vi "Active Graphic On Click.vi"(8 "error in (no error)":errorcluster, 10 "MousePoint":cluster{"x":i16, "y":i16}, 11 "Canvas in":refnum<class "Canvas.lvclass">) -> (0 "error out":errorcluster, 2 "Find?":bool, 3 "Canvas out":refnum<class "Canvas.lvclass">)   [LabVIEW 2015, in "Canvas.lvclass"]
uses:
  Canvas.lvclass
  Canvas.lvclass/Canvas.ctl
  Graphic/Graphic.lvclass
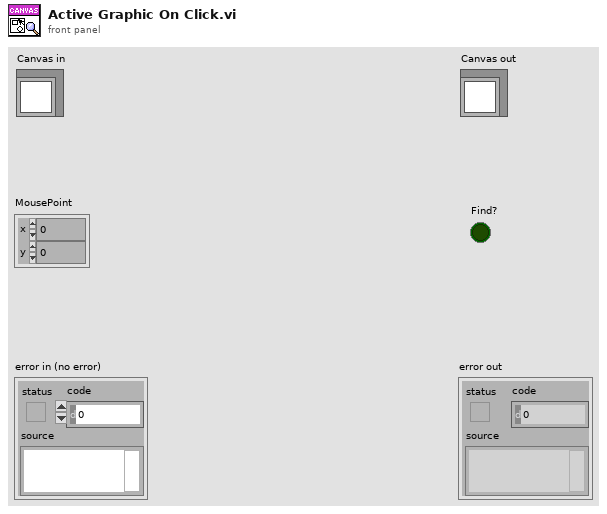
[diagram p1: front panel]
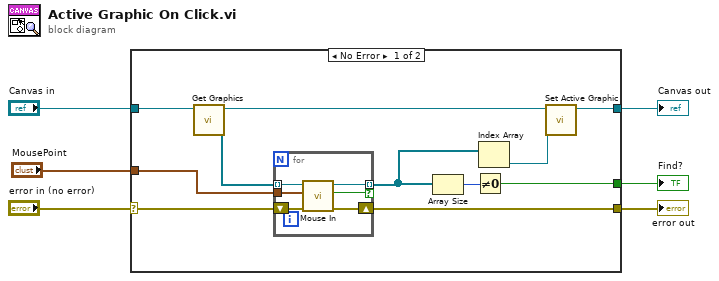
[diagram p0: block diagram]
diagram:
  n1 = case shown="No Error" "error in (no error)" {
    selector: "error in (no error)" -> [w13 w25]
    tunnel: [w12 w25] -> w5
    tunnel: [w8 w24] -> w3
    tunnel: "Canvas in" -> [w17 w24]
    tunnel: "MousePoint" -> [w14 _]
    tunnel: [w9 _] -> w1
    frame No Error {
      n2 = call "Get Graphics.vi"("Canvas in"=w17) -> ("Graphics"=w15:refnum<class "Graphic.lvclass">[], "Canvas out"=w16:refnum<class "Canvas.lvclass">)  [unwired: 8 in, 1 out]
      n3 = for {
        tunnel: w15 -> [w23] mode=indexing
        tunnel: w14 -> [w22]
        shift-right: [w20] -> w12
        shift-left: w13 -> [w21]
        tunnel: [w19] -> w11 mode=indexing if=w18
        n4 = call-dynamic "Mouse In.vi"("error in (no error)"=w21, "MousePoint"=w22, "Graphic in"=w23) -> ("error out"=w20:errorcluster, "In?"=w18:bool, "Graphic out"=w19:refnum<class "Graphic.lvclass">)  [unwired: 6 in]
      }
      n5 = Array Size(array=w11) -> (size(s)=w10:i32)
      n6 = Not Equal To 0?(x=w10) -> (x != 0?=w9:bool)
      n7 = Index Array(array=w11) -> (element=w7:refnum<class "Graphic.lvclass">)  [unwired: 1 in]
      n8 = call "Set Active Graphic.vi"("Operate Graphic"=w7, "Canvas in"=w16) -> ("Canvas out"=w8:refnum<class "Canvas.lvclass">)  [unwired: 8 in, 1 out]
    }
    frame Error {
    }
  }
  "error out" <- w5
  "Canvas out" <- w3
  "Find?" <- w1
